vi "Time Slide and Interpolate.vi"(7 "Target t0":timestamp, 10 "Target dt":dbl, 11 "input waveform":waveform(dbl)) -> (3 "output waveform":waveform(dbl))   [LabVIEW 2018, in "Waveform Equalizer.lvlib"]
uses:
  Waveform Equalizer.lvlib
  Greater or Equal with Epsilon.vi
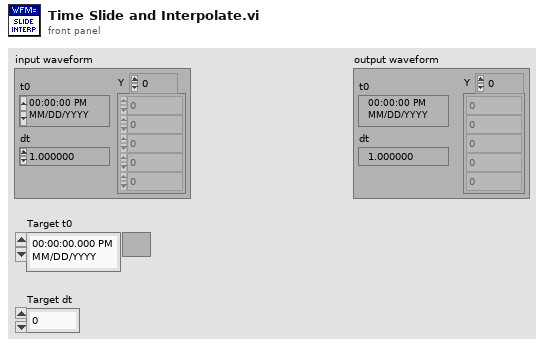
[diagram p1: front panel]
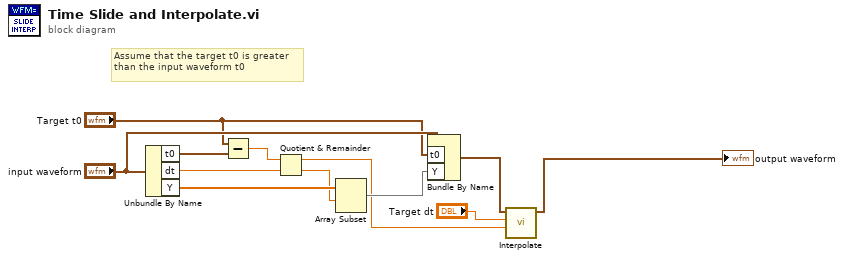
[diagram p0: block diagram]
diagram:
  # "Assume that the target t0 is greater than the input waveform t0"
  n1 = Unbundle By Name("input waveform") -> ("t0"=w12:timestamp, "dt"=w10:dbl, "Y"=w9:dbl[])
  n2 = Subtract(x="Target t0", y=w12) -> (x-y=w11:dbl)
  n3 = Quotient & Remainder(x=w11, y=w10) -> (x-y*floor(x/y)=w2:dbl, floor(x/y)=w8:dbl)
  n4 = Array Subset(array=w9, index=w8) -> (w6:dbl[])  [unwired: 1 in]
  n5 = Bundle By Name(cluster="input waveform", "t0"="Target t0", "Y"=w6) -> (w3:waveform(dbl))
  n6 = call "Interpolate.vi"("offset"=w2, "Target dt"="Target dt", "input waveform"=w3) -> ("output waveform"=→"output waveform":waveform(dbl))  [unwired: 8 in]
